vi "Arm.vi"(8 "error in (no error)":errorcluster, 10 "Arm":bool=TRUE, 11 "Measure Pulse in":refnum<class "Measure Pulse.lvclass">) -> (0 "error out":errorcluster, 3 "Measure Pulse out":refnum<class "Measure Pulse.lvclass">)   [LabVIEW 2015, in "Measure Pulse.lvclass"]
uses:
  Measure Pulse.lvclass
  Read Acquire Pulse Ref.vi
  Queued Listbox/Queued Listbox.xctl
  Common Measurements/Common Measurements.lvclass
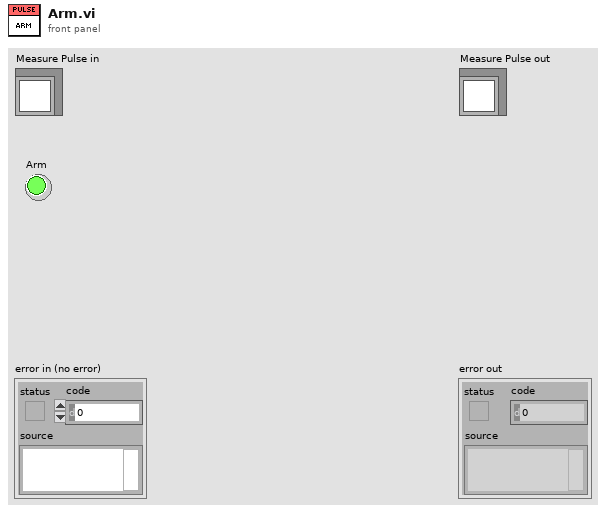
[diagram p1: front panel]
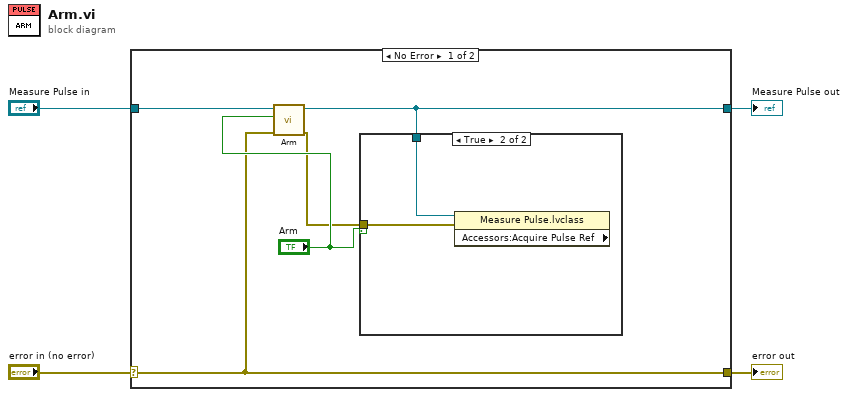
[diagram p0: block diagram]
diagram:
  n1 = case shown="No Error" "error in (no error)" {
    selector: "error in (no error)" -> [w6 w13]
    tunnel: [w6 w13] -> w3
    tunnel: [w8 w12] -> w1
    tunnel: "Measure Pulse in" -> [w9 w12]
    frame No Error {
      n2 = call-parent "Arm.vi"("error in (no error)"=w6, "Arm"="Arm", "Mag Lab Measurement in"=w9) -> ("error out"=w5:errorcluster, "Mag Lab Measurement out"=w8:refnum<class "Measure Pulse.lvclass">)  [unwired: 7 in]
      n3 = case shown="True" "Arm" {
        tunnel: w8 -> [_ w11]
        tunnel: w5 -> [_ w10]
        frame False {
        }
        frame True {
          n4 = property class="Measure Pulse.lvclass" props=["Accessors:Acquire Pulse Ref"](reference=w11, error in=w10) -> ()  [unwired: 3 out]
        }
      }
    }
    frame Error {
    }
  }
  "error out" <- w3
  "Measure Pulse out" <- w1
